vi "Read Test Group Data.vi"(8 "error in (no error)":errorcluster, 11 "Test Group in":refnum<class "Test Group.lvclass">) -> (0 "error out":errorcluster, 2 "Test Group Data":T1, 3 "Test Group out":refnum<class "Test Group.lvclass">)   [LabVIEW 2016, in "Test Group Manager.lvlib" / "Test Group.lvclass"]
uses:
  Test Group.lvclass
  Test Group.lvclass/Test Group.ctl
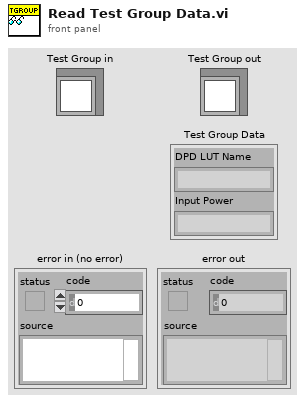
[diagram p1: front panel]
types:
  T1 = cluster{"DPD LUT Name":string, "Input Power":string}
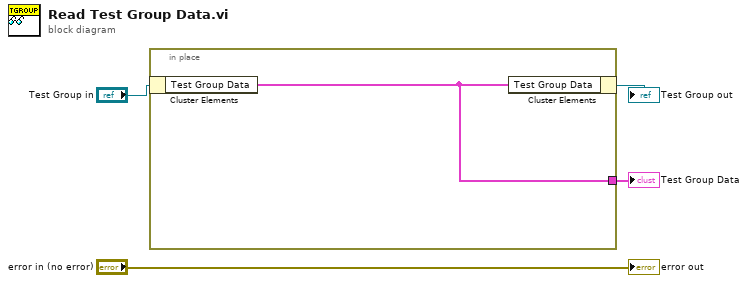
[diagram p0: block diagram]
diagram:
  n1 = in-place {
    in-place-border: [w5] -> w1
    n2 = in-place-cluster #1("Test Group in") -> ("Test Group Data"=w5:T1)
    n3 = in-place-cluster #1("Test Group Data"=w5) -> (→"Test Group out":refnum<class "Test Group.lvclass">)
  }
  "Test Group Data" <- w1
  "error out" <- "error in (no error)"
